vi "Module Main.vi"(8 "error in (no error)":errorcluster) -> (0 "error out":errorcluster)   [LabVIEW 2026, in "Control.lvlib"]
doc: "Module Main\nFor named purposes"
uses:
  Control.lvlib
  Private Control/Queue FGV Action.ctl
  User Event/User Event.lvlib
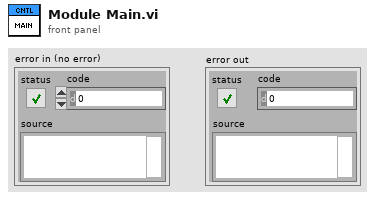
[diagram p1: front panel]
types:
  T1 = typedef "Control.lvlib/Queue FGV Action.ctl" = enum16{"Create", "Get", "Release"}
  T2 = typedef "Control.lvlib/Queue Element.ctl" = cluster{"Module Action":T3, "Data":variant}
  T3 = typedef "Control.lvlib/Module Action.ctl" = enum16{"Init", "Termination ", "Error", "Exit"}
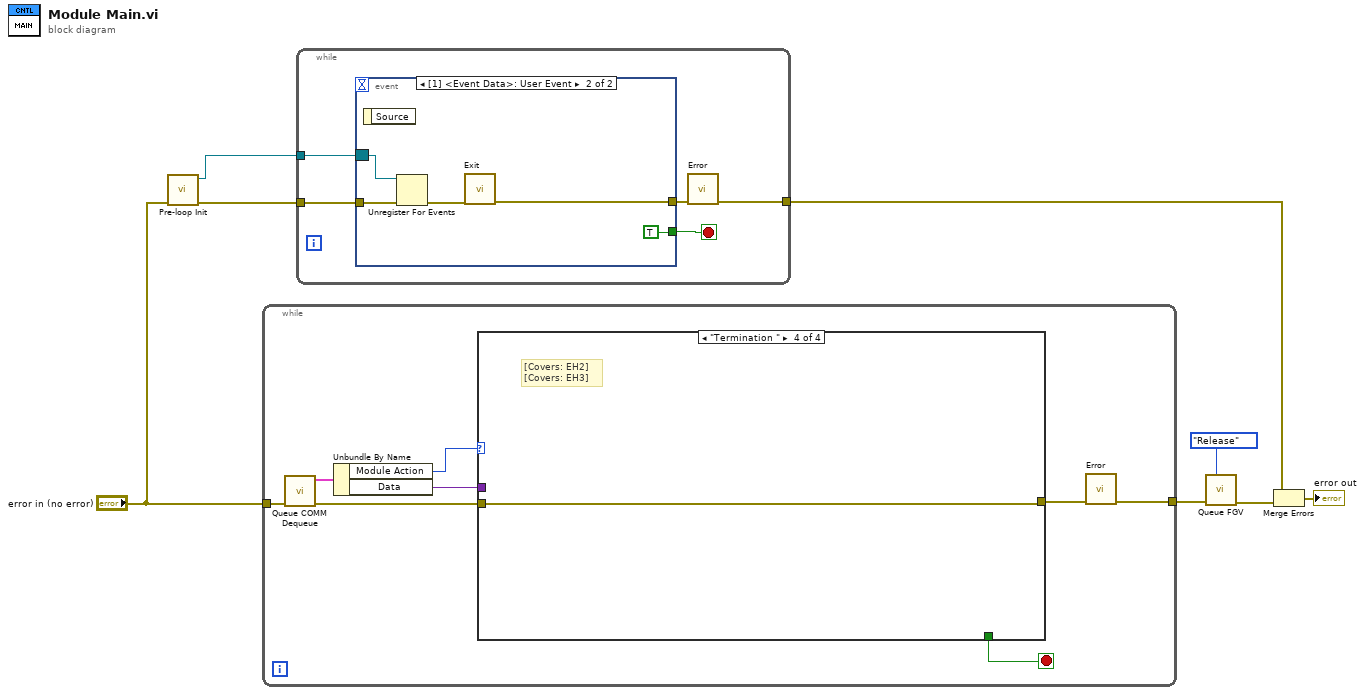
[diagram p0: block diagram]
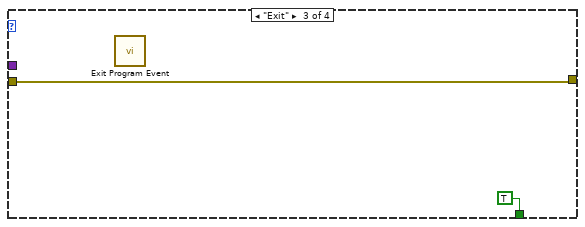
[diagram p4: hidden frame]
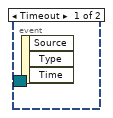
[diagram p5: hidden frame]
diagram:
  n1 = call "Pre-loop Init.vi"("error in (no error)"="error in (no error)") -> ("error out"=w7:errorcluster, "Event Registration Refnum"=w8:refnum<event-registration>)  [unwired: 9 in]
  n2 = while {
    tunnel: "error in (no error)" -> [w16]
    tunnel: [w10] -> w3
    stop <- w9 stop-if-true
    n3 = call "Queue COMM Dequeue.vi"("error in (no error)"=w16) -> ("error out"=w14:errorcluster, "element"=w15:T2)  [unwired: 9 in]
    n4 = Unbundle By Name(w15) -> ("Module Action"=w13:T3, "Data"=w12:variant)
    n5 = case shown="\"Termination \"" w13 {
      tunnel: w14 -> [w17 w18 w20 w21]
      tunnel: w12 -> [_ _ _ _]
      tunnel: [w17 w18 w20 w21] -> w11
      tunnel: [_ _ TRUE _] -> w9
      frame "Init", Default {
      }
      frame "Error" {
      }
      frame "Exit" {
        n6 = call "Exit Program Event.vi"() -> ()  [unwired: 11 in, 1 out]
      }
      frame "Termination " {
        # "[Covers: EH2] \n[Covers: EH3]"
      }
    }
    n7 = call "Error.vi"("error in (no error)"=w11) -> ("error out"=w10:errorcluster)  [unwired: 10 in]
  }
  n8 = while {
    tunnel: w8 -> [w26]
    tunnel: w7 -> [w25]
    tunnel: [w23] -> w5
    stop <- w22 stop-if-true
    n9 = event shown="[1] <Event Data>: User Event" {
      selector: w26 -> [_ w30]
      dyn-events: _ -> [_ _]
      timeout: _ -> [_ _]
      tunnel: w25 -> [_ w31]
      tunnel: [_ w28] -> w24
      tunnel: [_ TRUE] -> w22
      event Timeout {
        n10 = event-data() -> ()  [unwired: 1 in, 3 out]
      }
      event User Event {
        n11 = event-data() -> ()  [unwired: 1 in, 1 out]
        n12 = Unregister For Events(event registration refnum=w30, error in=w31) -> (error out=w29:errorcluster)
        n13 = call "Exit.vi"("error in (no error)"=w29) -> ("error out"=w28:errorcluster)  [unwired: 10 in]
      }
    }
    n14 = call "Error.vi"("error in (no error)"=w24) -> ("error out"=w23:errorcluster)  [unwired: 10 in]
  }
  n15 = call "Queue FGV.vi"("error in (no error)"=w3, "Queue FGV  Action"=Queue_FGV_Action."Release") -> ("error out"=w2:errorcluster)  [unwired: 8 in, 1 out]
  n16 = Merge Errors(w5, w2) -> (→"error out":errorcluster)
